vi "test - multiline Key.vi"(8 "error in (no error)":errorcluster, 11 "TestCase in":refnum<class "labview-config-library.lvclass">) -> (0 "error out":errorcluster, 3 "TestCase out":refnum<class "labview-config-library.lvclass">)   [LabVIEW 2017, in "labview-config-library.lvclass"]
uses:
  labview-config-library.lvclass
  <vilib>/addons/_JKI Toolkits/VI Tester/TestCase.llb/TestCase.lvclass
  C:/Program Files (x86)/National Instruments/LabVIEW 2017/vi.lib/addons/_JKI Toolkits/VI Tester/TestCase.llb/TestCase.lvclass
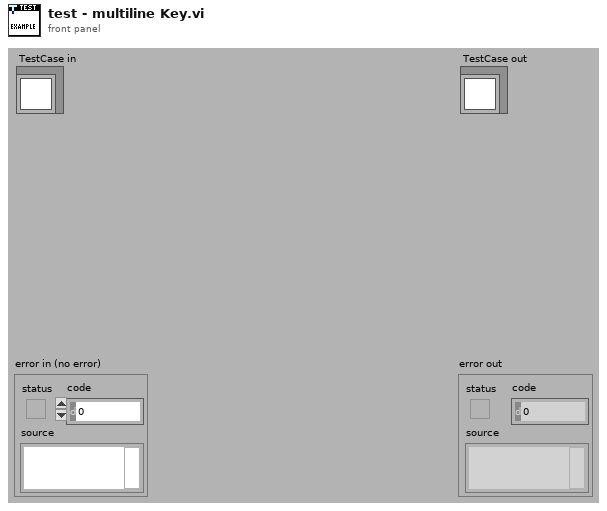
[diagram p1: front panel]
types:
  T1 = cluster{"Section Names":string[], "Key Names":string[], "Config":cluster{"String":string, "Boolean":bool, "Int":i32, "Uint":u32, "Float":dbl, "Raw":string}, string}
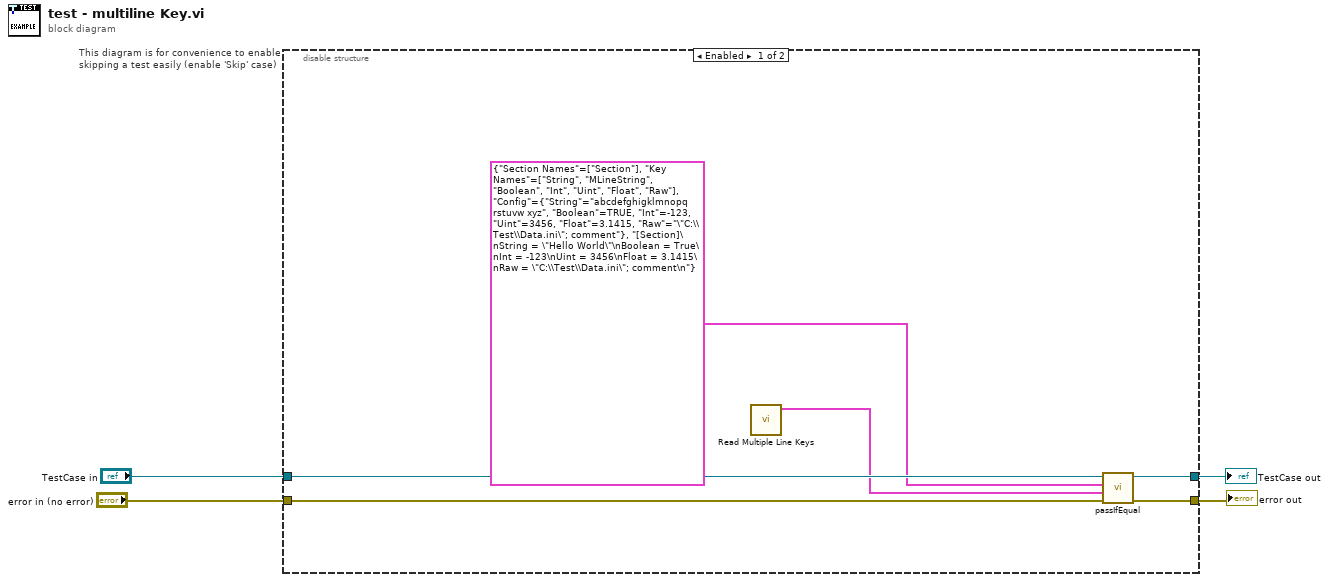
[diagram p0: block diagram]
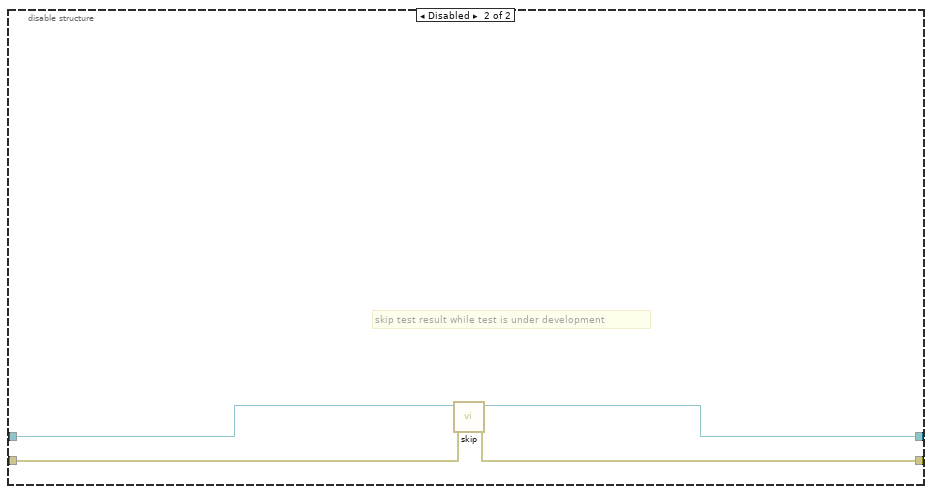
[diagram p2: hidden frame]
diagram:
  n1 = disable-structure "This diagram is for convenience to enable skipping a test easily (enable 'Skip' case)" shown="Enabled" {
    disable-tunnel: "TestCase in" -> [w10 w14]
    disable-tunnel: [w9 w12] -> w1
    disable-tunnel: [w8 w13] -> w3
    disable-tunnel: "error in (no error)" -> [w7 w11]
    frame Enabled {
      n2 = call "Read Multiple Line Keys.vi"() -> ("output cluster"=w6:T1)  [unwired: 10 in, 1 out]
      n3 = call-dynamic "passIfEqual.vi"("error in (no error)"=w7, "y"=w6, "x"=T1 {"Section Names"=["Section"], "Key Names"=["String", "MLineString", "Boolean", "Int", "Uint", "Float", "Raw"], "Config"={"String"="abcdefghigklmnopq rstuvw xyz", "Boolean"=TRUE, "Int"=-123, "Uint"=3456, "Float"=3.1415, "Raw"="\"C:\\Test\\Data.ini\"; comment"}, "[Section]\nString = \"Hello World\"\nBoolean = True\nInt = -123\nUint = 3456\nFloat = 3.1415\nRaw = \"C:\\Test\\Data.ini\"; comment\n"} ("output cluster"), "TestCase in"=w10) -> ("error out"=w8:errorcluster, "TestCase out"=w9:refnum<class "labview-config-library.lvclass">)  [unwired: 6 in]
    }
    frame Disabled {
      # "skip test result while test is under development"
      n4 = call <vilib>:"skip.vi"("error in (no error)"=w11, "TestCase in"=w14) -> ("error out"=w13:errorcluster, "TestCase out"=w12:refnum<class "labview-config-library.lvclass">)  [unwired: 8 in]
    }
  }
  "error out" <- w3
  "TestCase out" <- w1
